vi "Move Objects.vi"(11 "cluster in":T1) -> (3 "cluster out":T1)   [LabVIEW 2025]
uses:
  bd.ctl
  Node/Node.lvclass
  wire.ctl
  MultiDiagramStructure/MultiDiagramStructure.lvclass
  <vilib>/Utility/miscctls.llb/LVPositionTypeDef.ctl
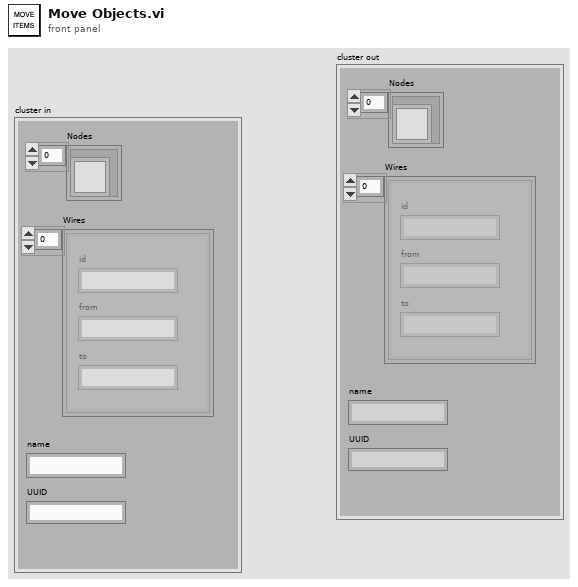
[diagram p1: front panel]
types:
  T1 = typedef "bd.ctl" = cluster{"Nodes":refnum<class "Node.lvclass">[], "Wires":T2[], "name":string, "UUID":string}
  T2 = typedef "wire.ctl" = cluster{"id":string, "from":string, "to":string}
  T3 = typedef "LVPositionTypeDef.ctl" = cluster{"Left":i32, "Top":i32}
  T4 = typedef "Subdiagram.ctl" = cluster{"diagram":refnum<vi>, "selector":string, "uuid":string}
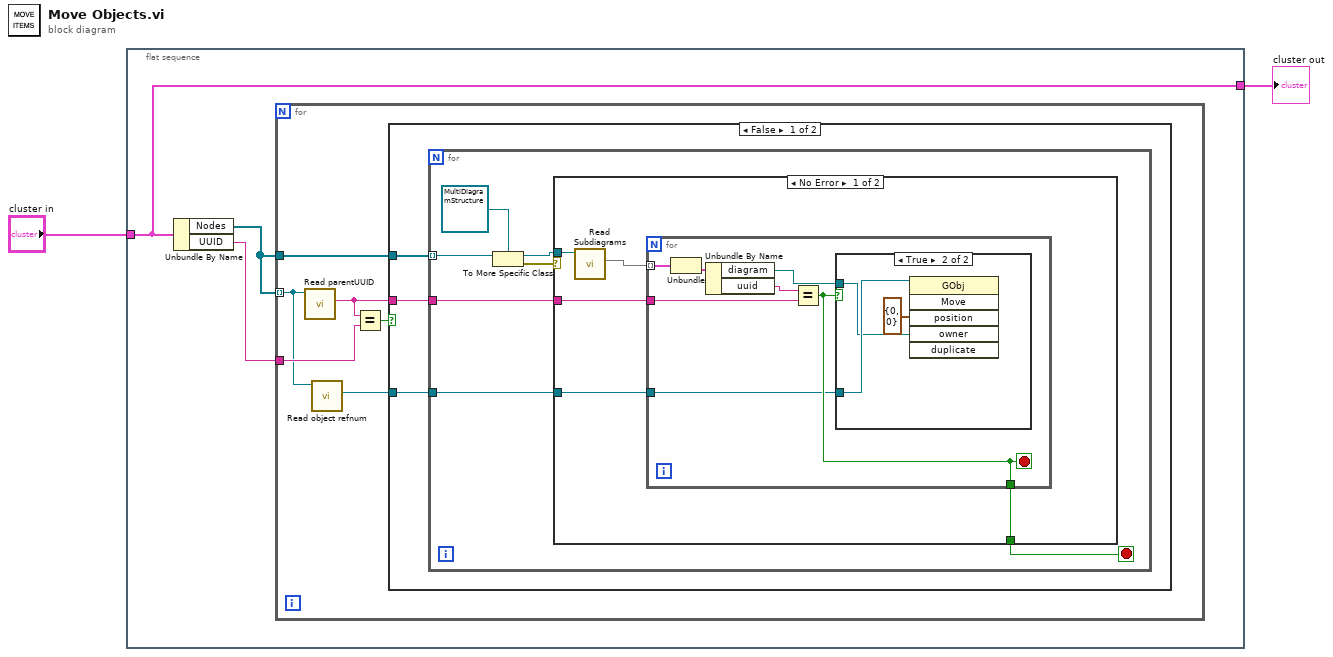
[diagram p0: block diagram]
diagram:
  n1 = flat-sequence {
    tunnel: "cluster in" -> [w3]
    tunnel: [w3] -> w1
    frame #0 {
      n2 = Unbundle By Name(w3) -> ("Nodes"=w5:refnum<class "Node.lvclass">[], "UUID"=w4:string)
      n3 = for {
        tunnel: w5 -> [w7] mode=indexing
        tunnel: w4 -> [w11]
        tunnel: w5 -> [w9]
        n4 = call-dynamic "Read parentUUID.vi"("Node in"=w7) -> ("parentUUID"=w8:string)  [unwired: 8 in, 2 out]
        n5 = call-dynamic "Read object refnum.vi"("Node in"=w7) -> ("object refnum"=w6:refnum<vi>)  [unwired: 8 in, 2 out]
        n6 = Equal?(x=w8, y=w11) -> (x = y?=w10:bool)
        n7 = case shown="False" w10 {
          tunnel: w9 -> [w14 _]
          tunnel: w8 -> [w13 _]
          tunnel: w6 -> [w12 _]
          frame False {
            n8 = for {
              tunnel: w14 -> [w21] mode=indexing
              tunnel: w13 -> [w17]
              tunnel: w12 -> [w15]
              stop <- w16 stop-if-true
              n9 = To More Specific Class(target class=refnum<class "MultiDiagramStructure.lvclass"> refnum ("MultiDiagramStructure.lvclass"), reference=w21) -> (specific class reference=w18:refnum<class "MultiDiagramStructure.lvclass">, error out=w19:errorcluster)  [unwired: 1 in]
              n10 = case shown="No Error" w19 {
                tunnel: w18 -> [w26 _]
                tunnel: w17 -> [w24 _]
                tunnel: [w23 _] -> w16
                tunnel: w15 -> [w22 _]
                frame No Error {
                  n11 = call-dynamic "Read Subdiagrams.vi"("MultiDiagramStructure in"=w26) -> ("Subdiagrams"=w25:map{u64, T4})  [unwired: 8 in, 2 out]
                  n12 = for {
                    tunnel: w25 -> [w33] mode=indexing
                    tunnel: w24 -> [w32]
                    tunnel: [w31] -> w23
                    tunnel: w22 -> [w30]
                    stop <- w31 stop-if-true
                    n13 = Unbundle(w33) -> ("Subdiagram"=w29:T4)  [unwired: 1 out]
                    n14 = Unbundle By Name(w29) -> ("diagram"=w28:refnum<vi>, "uuid"=w27:string)
                    n15 = Equal?(x=w27, y=w32) -> (x = y?=w31:bool)
                    n16 = case shown="True" w31 {
                      tunnel: w30 -> [_ w36]
                      tunnel: w28 -> [_ w35]
                      frame False {
                      }
                      frame True {
                        n17 = invoke class="GObj" method="Move"(reference=w36, "position"=T3 {"Left"=0, "Top"=0}, "owner"=w35) -> ()  [unwired: 3 in, 6 out]
                      }
                    }
                  }
                }
                frame Error {
                }
              }
            }
          }
          frame True {
          }
        }
      }
    }
  }
  "cluster out" <- w1
